vi "Count.vi"(8 "error in (no error)":errorcluster, 11 "ListImp in":refnum<class "ListImp.lvclass">) -> (0 "error out":errorcluster, 2 "Number of Items":i32, 3 "ListImp out":refnum<class "ListImp.lvclass">)   [LabVIEW 2013, in "LapDog.Collections.v_.Lists.lvlib" / "ListImp.lvclass"]
uses:
  ListImp.lvclass
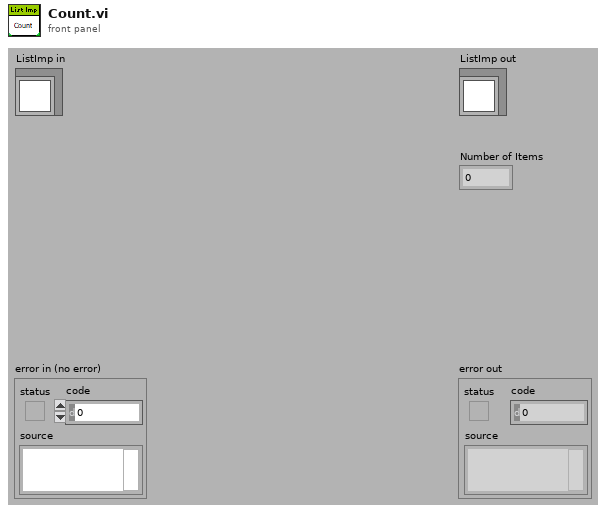
[diagram p1: front panel]
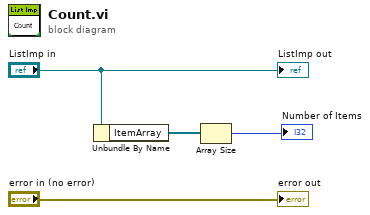
[diagram p0: block diagram]
diagram:
  n1 = Unbundle By Name("ListImp in") -> ("ItemArray"=w2:refnum<class>[])
  n2 = Array Size(array=w2) -> (size(s)=→"Number of Items":i32)
  "error out" <- "error in (no error)"
  "ListImp out" <- "ListImp in"
